vi "Auton PickUpTote Encoder.vi"() -> ()   [LabVIEW 2014]
uses:
  Robot Global Data.vi
panel:
  in  "Wait Time between each step":dbl=0.5
  out "Start Encoder position":dbl
  out "Current Step 2":string
  in  "Elevator to Raise Tote to carrying Height":dbl=50.0
  in  "Raise Elevator Power 2":dbl=0.8
  in  "Elevator Power 2":dbl=-0.8
  in  "Elevator to Tote1 drop distance 2":dbl=50.0
  in  "Elevator timeout 4":u32=1
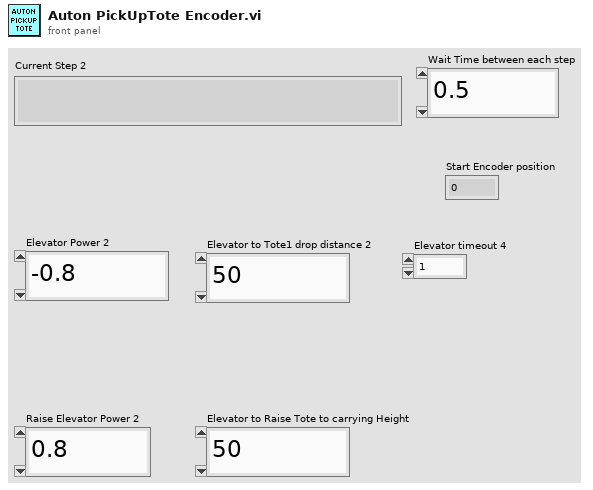
[diagram p1: front panel]
types:
  T1 = typedef "WPI_MotorControlDeviceRef.ctl" = cluster{"DeviceStatus":errorcluster, "Type":T2, "PWM":cluster{"Controller":T3, "PWM Channel":T4, "DeadBand":T5}, "CAN":cluster{"Device Number":u8, "Control Mode":T6, "Semaphore":T7, "Max Vout":dbl, "TalonSRX Control Mode":T8}, "Invert":bool, "TransformRef":T9, "InvTransformRef":T9}
  T2 = typedef "WPI_MotorControlType.ctl" = enum16{"PWM", "CAN", "CANTalonSRX"}
  T3 = typedef "FPGA_TypedefDigitalModule.ctl" = enum16{"Controller 1"}
  T4 = typedef "FPGA_DIOPWMChannel.ctl" = enum8{"PWM 0", "PWM 1", "PWM 2", "PWM 3", "PWM 4", "PWM 5", "PWM 6", "PWM 7", "PWM 8", "PWM 9", "PWM MXP 0", "PWM MXP 1", "PWM MXP 2", "PWM MXP 3", "PWM MXP 4", "PWM MXP 5", "PWM MXP 6", "PWM MXP 7", "PWM MXP 8", "PWM MXP 9", "Invalid"}
  T5 = typedef "WPI_PWMDeadband.ctl" = cluster{"Name":string, "maxPositivePwm":i32, "minPositivePwm":i32, "centerPwm":i32, "maxNegativePwm":i32, "minNegativePwm":i32, "angularRange":u16}
  T6 = typedef "WPI_CANJaguar_ControlMode.ctl" = enum8{"Percent VBus", "Current", "Speed", "Position", "Voltage"}
  T7 = typedef "Semaphore RefNum" = refnum<k1>
  T8 = typedef "WPI_CANTalonSRX_APIControlMode.ctl" = enum8{"Percent VBus", "Speed", "Position", "Slave", "Unchanged / Invalid"}
  T9 = typedef "WPI_PWMTransform_ConPane.ctl" = refnum<vi>
  T10 = typedef "WPI_EncoderDevRef.ctl" = cluster{"DevStatus":errorcluster, "EncoderIndex":T11, "CounterIndex":T12, "DistancePerCount":dbl, "Decoding Type":T13}
  T11 = typedef "FPGA_EncoderIdx.ctl" = enum8{"Enc 0", "Enc 1", "Enc 2", "Enc 3", "Enc 4", "Enc 5", "Enc 6", "Enc 7", "Invalid"}
  T12 = typedef "FPGA_CounterCtrSystemIndex.ctl" = enum8{"Ctr 0", "Ctr 1", "Ctr 2", "Ctr 3", "Ctr 4", "Ctr 5", "Ctr 6", "Ctr 7", "Invalid"}
  T13 = typedef "WPI_EncoderType.ctl" = enum16{"1x", "2x", "4x"}
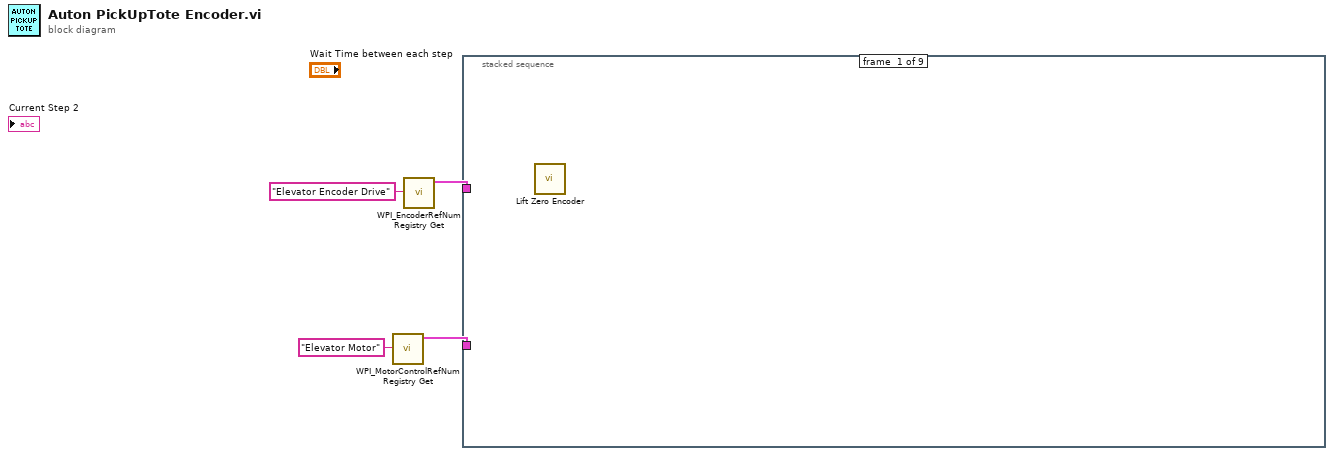
[diagram p0: block diagram]
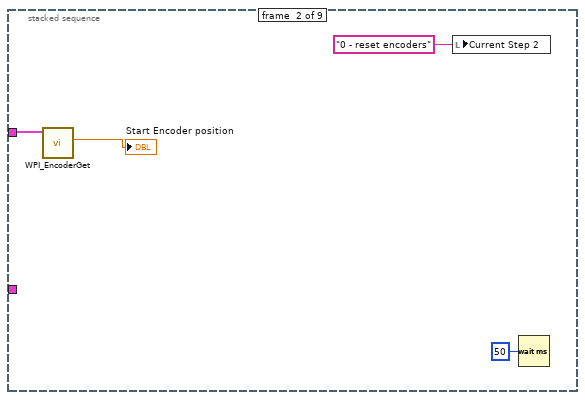
[diagram p2: hidden frame]
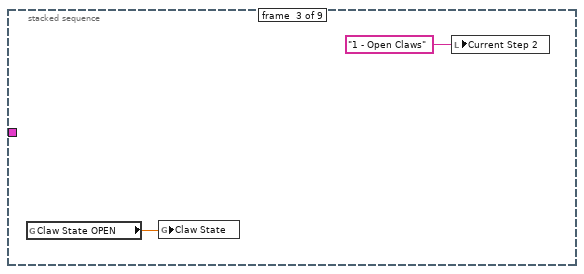
[diagram p3: hidden frame]
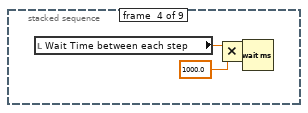
[diagram p4: hidden frame]
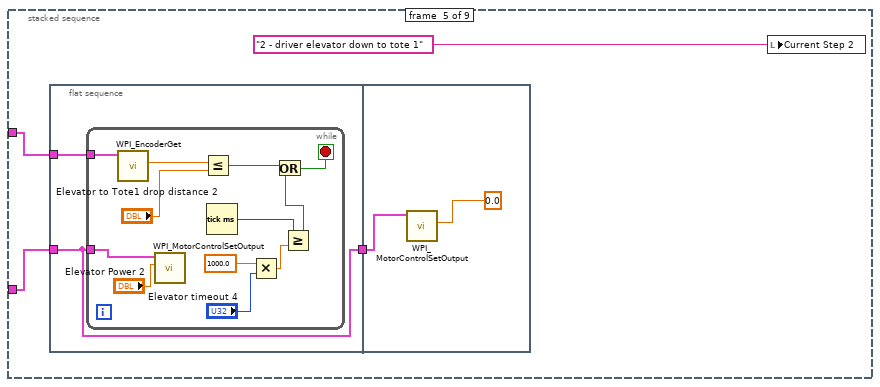
[diagram p5: hidden frame]
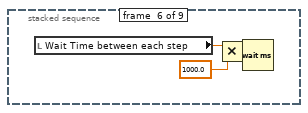
[diagram p6: hidden frame]
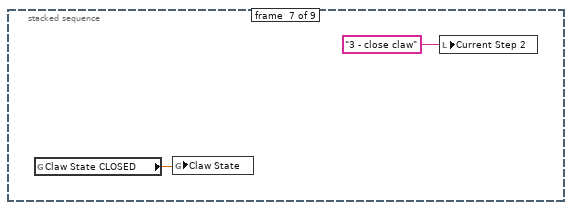
[diagram p7: hidden frame]
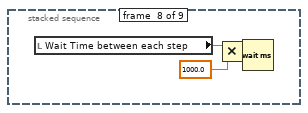
[diagram p8: hidden frame]
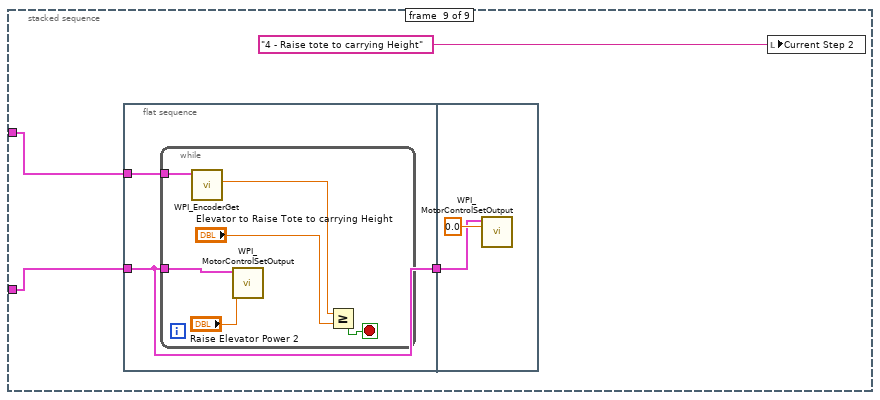
[diagram p9: hidden frame]
diagram:
  n1 = call <vilib>:"WPI_MotorControlRefNum Registry Get.vi"("refnum name"="Elevator Motor") -> ("MotorControlDevRef"=w1:T1)  [unwired: 9 in, 1 out]
  n2 = call <vilib>:"WPI_EncoderRefNum Registry Get.vi"("refnum name"="Elevator Encoder Drive") -> ("EncoderDevRef"=w3:T10)  [unwired: 9 in, 1 out]
  n3 = stacked-sequence {
    tunnel: w3 -> [_ w6 _ _ w15 _ _ _ w43]
    tunnel: w1 -> [_ _ _ _ w16 _ _ _ w44]
    frame #0 {
      n4 = call "Lift Zero Encoder.vi"() -> ()  [unwired: 12 in]
    }
    frame #1 {
      n5 = call <vilib>:"WPI_EncoderGet.vi"("EncoderDevRef"=w6) -> ("Distance"=→"Start Encoder position":dbl)  [unwired: 5 in, 5 out]
      n6 = local write "Current Step 2"("0 - reset encoders" ("Current Step")) -> ()
      n7 = Wait (ms)(milliseconds to wait=u32 50) -> ()  [unwired: 1 out]
    }
    frame #2 {
      n8 = global read "Robot Global Data.vi" "Claw State OPEN"() -> (w9:dbl)
      n9 = global write "Robot Global Data.vi" "Claw State"(w9) -> ()
      n10 = local write "Current Step 2"("1 - Open Claws" ("Current Step")) -> ()
    }
    frame #3 {
      n11 = local read "Wait Time between each step"() -> (w13:dbl)
      n12 = Multiply(x=w13, y=1000.0) -> (x*y=w12:dbl)
      n13 = Wait (ms)(milliseconds to wait=w12) -> ()  [unwired: 1 out]
    }
    frame #4 {
      n14 = flat-sequence {
        tunnel: w16 -> [w19]
        tunnel: [w19] -> w14
        tunnel: w15 -> [w18]
        tunnel: w14 -> [w33]
        frame #0 {
          n15 = while {
            tunnel: w19 -> [w31]
            tunnel: w18 -> [w30]
            stop <- w20 stop-if-true
            n16 = call <vilib>:"WPI_EncoderGet.vi"("EncoderDevRef"=w30) -> ("Distance"=w29:dbl)  [unwired: 5 in, 5 out]
            n17 = call <vilib>:"WPI_MotorControlSetOutput.vi"("Output"="Elevator Power 2", "MotorControlDevRef"=w31) -> ()  [unwired: 7 in, 3 out]
            n18 = Less Or Equal?(x=w29, y="Elevator to Tote1 drop distance 2") -> (x <= y?=w21:bool)
            n19 = Tick Count (ms)() -> (millisecond timer value=w26:u32)
            n20 = Multiply(x=1000.0, y="Elevator timeout 4") -> (x*y=w22:dbl)
            n21 = Greater Or Equal?(x=w26, y=w22) -> (x >= y?=w25:bool)
            n22 = Or(x=w21, y=w25) -> (x .or. y?=w20:bool)
          }
        }
        frame #1 {
          n23 = call <vilib>:"WPI_MotorControlSetOutput.vi"("Output"=0.0, "MotorControlDevRef"=w33) -> ()  [unwired: 7 in, 3 out]
        }
      }
      n24 = local write "Current Step 2"("2 - driver elevator down to tote 1" ("Current Step")) -> ()
    }
    frame #5 {
      n25 = local read "Wait Time between each step"() -> (w36:dbl)
      n26 = Multiply(x=w36, y=1000.0) -> (x*y=w35:dbl)
      n27 = Wait (ms)(milliseconds to wait=w35) -> ()  [unwired: 1 out]
    }
    frame #6 {
      n28 = global read "Robot Global Data.vi" "Claw State CLOSED"() -> (w37:dbl)
      n29 = global write "Robot Global Data.vi" "Claw State"(w37) -> ()
      n30 = local write "Current Step 2"("3 - close claw" ("Current Step")) -> ()
    }
    frame #7 {
      n31 = local read "Wait Time between each step"() -> (w41:dbl)
      n32 = Multiply(x=w41, y=1000.0) -> (x*y=w40:dbl)
      n33 = Wait (ms)(milliseconds to wait=w40) -> ()  [unwired: 1 out]
    }
    frame #8 {
      n34 = flat-sequence {
        tunnel: w44 -> [w47]
        tunnel: [w47] -> w42
        tunnel: w43 -> [w46]
        tunnel: w42 -> [w54]
        frame #0 {
          n35 = while {
            tunnel: w47 -> [w53]
            tunnel: w46 -> [w52]
            stop <- w51 stop-if-true
            n36 = call <vilib>:"WPI_EncoderGet.vi"("EncoderDevRef"=w52) -> ("Distance"=w50:dbl)  [unwired: 5 in, 5 out]
            n37 = call <vilib>:"WPI_MotorControlSetOutput.vi"("Output"="Raise Elevator Power 2", "MotorControlDevRef"=w53) -> ()  [unwired: 7 in, 3 out]
            n38 = Greater Or Equal?(x=w50, y="Elevator to Raise Tote to carrying Height") -> (x >= y?=w51:bool)
          }
        }
        frame #1 {
          n39 = call <vilib>:"WPI_MotorControlSetOutput.vi"("Output"=0.0, "MotorControlDevRef"=w54) -> ()  [unwired: 7 in, 3 out]
        }
      }
      n40 = local write "Current Step 2"("4 - Raise tote to carrying Height" ("Current Step")) -> ()
    }
  }
